vi "PCO_SetStorageMode.vi"(8 "error in (no error)":errorcluster {"code" format="%x"}, 10 "wStorageMode":u16(ring) items=["recorder", "FIFO buffer"], 11 "ph":u64) -> (0 "error out":errorcluster {"code" format="%x"}, 2 "ErrorMessage":i32 format="%x", 3 "ph out":u64)   [LabVIEW 2019, in "SDK.lvlib" / "RecordingControl.lvlib"]
doc: "<b>Description:</b>\nThis function does set the storage mode of the camera.\nStorage mode can be set to either [recorder] or [FIFO buffer] mode.\n\n<b>-->StorageMode [recorder]</b>\n Images are recorded and stored in the current selected segment of the camera internal memory (CamRAM)\nIf PCO_SetRecorderSubmode is [sequence] recording is stopped, when the last buffer in the segment is reached\nIf PCO_SetRecorderSubmode is [ring buffer] the oldest image is overwritten, when the segment is full\nWhile PCO_SetRecordingState is [run] the most recent image is transferred on an image request\nWhen PCO_SetRecordingState is [stop] the recorded images can be readout from the camera memory using an image number index. Image number 1 is always the oldest image in the segment\n\n<b>-->StorageMode [FIFO buffer]</b>\nCamera internal memory (CamRAM) is used as huge FIFO buffer to bypass short bottlenecks in data transmission\nIf buffer overflows, the oldest images are overwritten\nWhile PCO_SetRecordingState is [run] the oldest image is transferred on an image request\nWhen PCO_SetRecordingState is [stop] the recorded and not already transferred images can be read from the camera memory using an image number index. Image number 1 is always the oldest image in the segment\nNo PCO_SetRecorderSubmode available\n\n<b>Supported camera type:</b>\npco.dimax, pco.pixelfly usb, pco.ultraviolet, pco.1200, pco.1300, pco.1400, pco.1600, pco.2000, pco.4000\n\n<b>Descriptor dependency:</b>\nNone"
uses:
  RecordingControl.lvlib
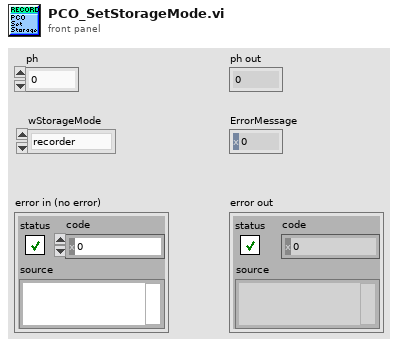
[diagram p1: front panel]
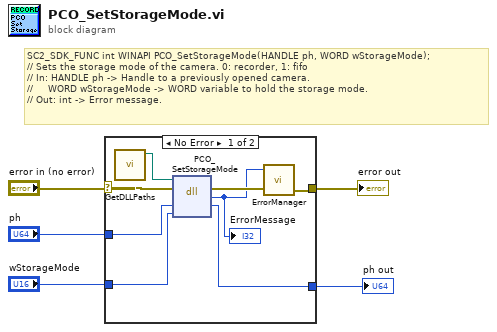
[diagram p0: block diagram]
diagram:
  # "SC2_SDK_FUNC int WINAPI PCO_SetStorageMode(HANDLE ph, WORD wStorageMode);\n// Sets the storage mode of the camera. 0: recorder, 1: fifo\n// In: HANDLE ph -> Handle to a previously opened camera.\n//     WORD wStorageMode -> WORD variable to hold the storage mode.\n// Out: int -> Error message."
  n1 = case shown="No Error" "error in (no error)" {
    selector: "error in (no error)" -> [w10 w15]
    tunnel: "ph" -> [w13 w14]
    tunnel: [w12 w14] -> w4
    tunnel: "wStorageMode" -> [w11 _]
    tunnel: [w8 w15] -> w2
    frame No Error {
      n2 = call "GetDLLPaths.vi"() -> ("SC2_Cam_Path"=w6:path)  [unwired: 8 in, 3 out]
      n3 = dll-call lib="?" fn="PCO_SetStorageMode"(path in=w6, error in=w10, "ph"=w13, "wStorageMode"=w11) -> (error out=w9:errorcluster, "return type"=w7:i32, "ph"=w12:u64)  [unwired: 2 in, 1 out]
      "ErrorMessage" <- w7
      n4 = call "ErrorManager.vi"("error in (no error)"=w9, "error code"=w7) -> ("error out"=w8:errorcluster)  [unwired: 2 in, 1 out]
    }
    frame Error {
    }
  }
  "ph out" <- w4
  "error out" <- w2
